vi "Measure Delay for Active and Idle Channels.vi"(7 "tolerance":dbl=0.1 format="%#_13g", 8 "error in (no error)":errorcluster, 9 "maximum delay":i32, 10 "waveforms subset":waveform(dbl)[](array[waveform]), 11 "alignment reference signal":waveform(dbl)) -> (0 "error out":errorcluster, 1 "delays [s]":dbl[](array[numeric]), 2 "waveforms subset dup":waveform(dbl)[](array[waveform]), 3 "reference detected":bool)   [LabVIEW 2022 SP3]
doc: "This VI measures the delay on all channels based on alignment reference signal. For channels with low coherence with alignment reference signal, channel delay is adjusted to match a high coherence channel."
uses:
  <vilib>/addons/_NISVFA/_Shared subVIs/Common/svc_Check for Waveform Parameter Continuity (N Ch).vi
  <vilib>/addons/Sound and Vibration/svt_Calibration/SV Measure Delay and Polarity and Coherence.vi
  <vilib>/addons/_NISVFA/_Shared subVIs/Common/sv_Get NI Property Name String.vi
  <vilib>/addons/_NISVFA/_Shared subVIs/Common/svc_Check for Waveform Parameter Continuity (no state).vi
  <vilib>/Analysis/_algsub.llb/Vector Norm.vi
  <vilib>/Analysis/_algsub.llb/Real Vector Norm.vi
  <vilib>/addons/_NISVFA/_Shared subVIs/Common/SV Get Data Subset.vi
  <vilib>/addons/_NISVFA/_Shared subVIs/Common/svc_Get Array Subset (Index).vi
  <vilib>/addons/_NISVFA/_Shared subVIs/Common/svc_Get SV Channel Info.vi
  <vilib>/addons/_NISVFA/_Shared subVIs/Common/svc_Coerce Index and Length.vi
  <vilib>/addons/_NISVFA/_Shared subVIs/Common/svc_Unit Label to Engineering Units.vi
  <vilib>/addons/_NISVFA/_Shared subVIs/Common/svc_Engineering Units to Unit Label.vi
  <vilib>/addons/_NISVFA/_Shared subVIs/Common/svc_Conditional Merge Error.vi
  <vilib>/measure/maresamp.llb/Resample Waveforms (single shot).vi
  <vilib>/measure/maresamp.llb/Resample Waveform (single shot).vi
  <vilib>/addons/_NISVFA/_Shared subVIs/Common/svc_Check dt for Equal Sample Rates.vi
  <vilib>/Waveform/TSOps.llb/Timestamp Subtract.vi
  <vilib>/Analysis/2dsp.llb/CrossCorrelation.vi
  <vilib>/Analysis/2dsp.llb/1D Cross Correlation (DBL).vi
  <vilib>/addons/_NISVFA/_Shared subVIs/Common/svc_Fit Quadratic to Max Three Points in Array.vi
  <vilib>/Utility/error.llb/Error Cluster From Error Code.vi
  <vilib>/addons/_NISVFA/_Shared subVIs/Common/svc_Caller VI Returned in Error Source.vi
  <vilib>/addons/Sound and Vibration/svt_Calibration/SoundVib_Calibration.lvlib
  Program Files/NI/LVAddons/nisvt/1/examples/Sound and Vibration/SoundVib_Audio Examples.lvlib
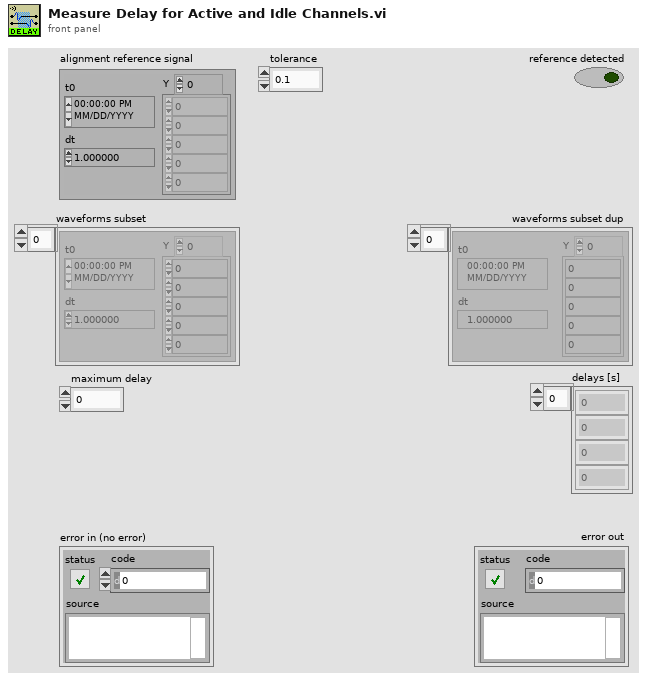
[diagram p1: front panel]
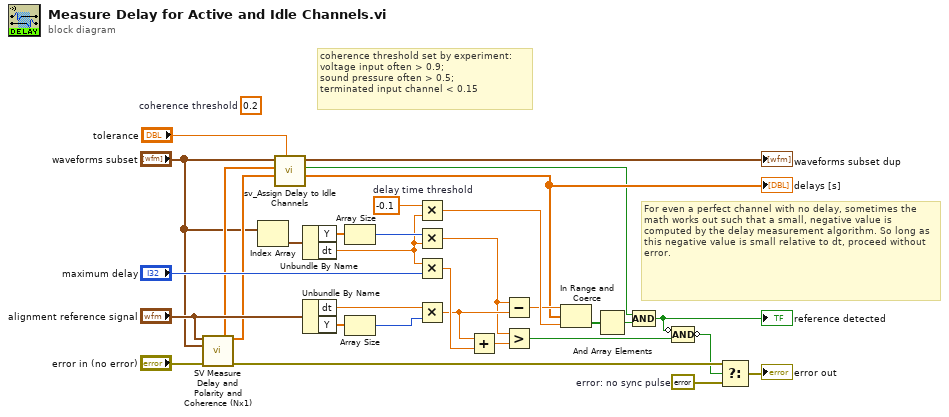
[diagram p0: block diagram]
diagram:
  (unwired) 0.2  # coherence threshold
  w19 = errorcluster {"status"=TRUE, "code"=-1984, "source"="alignment. Sync pulse not detected. Verify configuration and wiring."}  # error: no sync pulse
  w29 = -0.1  # delay time threshold
  # "For even a perfect channel with no delay, sometimes the math works out such that a small, negative value is computed by the delay measurement algorithm. So long as this negative value is small relative to dt, proceed without error."
  # "coherence threshold set by experiment: \nvoltage input often > 0.9;  \nsound pressure often > 0.5;  \nterminated input channel < 0.15"
  n1 = call <vilib>:"SV Measure Delay and Polarity and Coherence (Nx1).vi"("reference signal"="alignment reference signal", "response signals"="waveforms subset", "error in"="error in (no error)") -> ("coherences"=w4:dbl[], "delays [s]"=w5:dbl[], "error out"=w18:errorcluster)  [unwired: 8 in, 2 out]
  n2 = Index Array(array="waveforms subset") -> (element=w22:waveform(dbl))  [unwired: 1 in]
  n3 = call "sv_Assign Delay to Idle Channels.vi"("tolerance"="tolerance", "delays [s] in"=w5, "coherences"=w4, "acquired responses"="waveforms subset") -> ("delays [s] out"=w7:dbl[], "verified"=w6:bool, "acquired responses dup"=→"waveforms subset dup":waveform(dbl)[])  [unwired: 5 in]
  "delays [s]" <- w7
  n4 = Unbundle By Name ("Get Waveform Components")(w22) -> ("Y"=w31:dbl[], "dt"=w13:dbl)
  n5 = Unbundle By Name ("Get Waveform Components")("alignment reference signal") -> ("dt"=w23:dbl, "Y"=w20:dbl[])
  n6 = Array Size(array=w31) -> (size(s)=w32:i32)
  n7 = Array Size(array=w20) -> (size(s)=w24:i32)
  n8 = Multiply(x=w29, y=w13) -> (x*y=w12:dbl)
  n9 = Multiply(x=w32, y=w13) -> (x*y=w2:dbl)
  n10 = Multiply(x=w13, y="maximum delay") -> (x*y=w26:dbl)
  n11 = Multiply(x=w23, y=w24) -> (x*y=w11:dbl)
  n12 = Add(x=w11, y=w26) -> (x+y=w28:dbl)
  n13 = Subtract(x=w2, y=w11) -> (x-y=w10:dbl)
  n14 = Greater?(x=w2, y=w28) -> (0:w17:bool)
  n15 = In Range and Coerce(upper limit=w10, x=w7, lower limit=w12) -> (In Range?=w9:bool[])  [unwired: 1 out]
  n16 = And Array Elements(Boolean array=w9) -> (logical AND=w27:bool)
  n17 = Compound Arithmetic op=AND(w6, w27) -> (w16:bool)
  "reference detected" <- w16
  n18 = Compound Arithmetic op=AND(invert w16, w17) -> (invert w15:bool)
  n19 = Select(t=w18, s=w15, f=w19) -> (s? t:f=→"error out":errorcluster)
